vi "ex3-3.vi"() -> ()   [LabVIEW 2009]
panel:
  out "迴圈執行次數":i32
  out "X+Y":dbl
  in  "Y":dbl
  in  "X":dbl
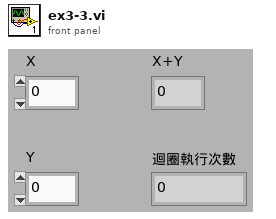
[diagram p1: front panel]
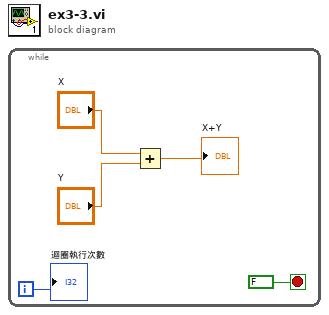
[diagram p0: block diagram]
diagram:
  n1 = while {
    i -> [w1]
    stop <- FALSE stop-if-true
    n2 = Add(x="X", y="Y") -> (x+y=→"X+Y":dbl)
    "迴圈執行次數" <- w1
  }
